vi "Angle_1.vi"() -> ()   [LabVIEW 2020]
uses:
  Support/Controls/Cmd_Mouse Popup.ctl
  Support/Controls/Clst_Initialize Input.ctl
  Support/Controls/Cmd_Var Data IO.ctl
  Variables/Global_Cal Info.vi
  Support/Public/Polymorph/Input Check_TBL.vi
  Support/Public/Polymorph/Input Check_TextBox.vi
panel:
  in  "반지름":string caption="투영면 반지름 (mm)"
  out "최소범위":string
  out "STD set":string[][](table) caption="○ 기준기 조합 (값)"
  in  "Measured 2":string[][](table)
  in  "표시방식":string(combo)
  out "단위":string
  out "최대범위":string
  in  "Spec 변경":bool
  in  "Random":bool
  out "Resolution":string[][](table) caption="Spec"
  out "Spec":string[][](table)
  out "제목":string
  out "에러 출력":errorcluster
  out "Condition":string[][](table) caption="2. 직선성 시험"
  in  "최소눈금":string(combo)
  in  "Measured":string[][](table) caption="저울의 지시값"
  out "Load?":bool
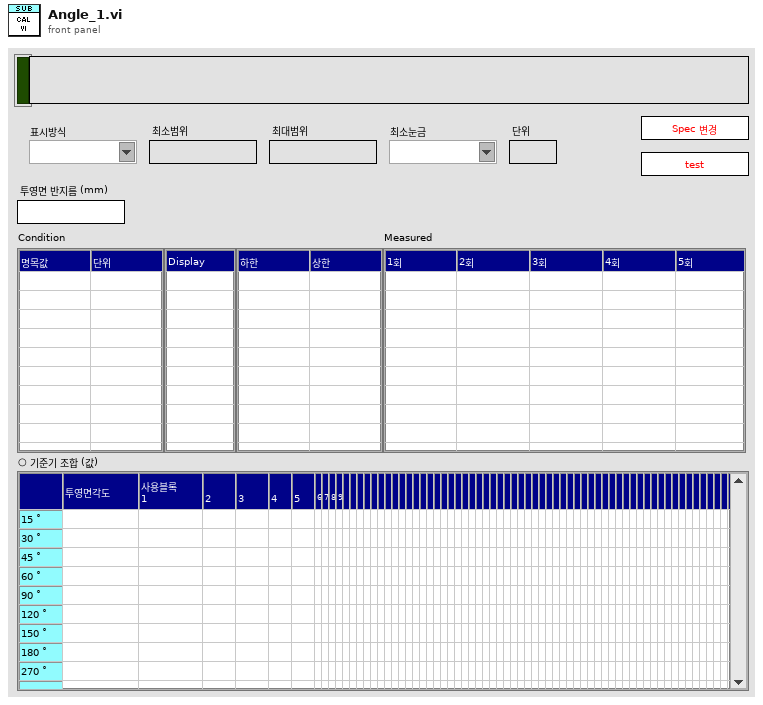
[diagram p1: front panel]
types:
  T1 = typedef "Cmd_Mouse Popup.ctl" = enum16{"활성화", "메뉴선택"}
  T2 = cluster{"Shift":bool, "Ctrl":bool, "Alt":bool, "Cmd":bool, "Opt":bool}
  T3 = typedef "Clst_Initialize Input.ctl" = cluster{"Initialize 1":cluster{"Condition":refnum<vi>[], "Spec":refnum<vi>[], "Measured":refnum<vi>[], "Resolution":refnum<vi>[], "Func_ext":string, "제목":refnum<vi>, "Measured_ADJ":refnum<vi>[]}, "Initialize 2":cluster{"문자열":refnum<vi>[], "콤보박스":refnum<vi>[], "링":refnum<vi>[], "열거형":refnum<vi>[], "테이블":refnum<vi>[], "여러열":refnum<vi>[], "디지털(DBL)":refnum<vi>[], "3D string":refnum<vi>[], "ctrl":refnum<vi>[], "boolean":refnum<vi>[]}}
  T4 = typedef "Cmd_Var Data IO.ctl" = enum16{"Condition", "Condition Default", "Condition_Temp", "Resolution", "Resolution Default", "Resolution Old", "Spec", "Spec Default", "Spec Old", "Spec Temp", "Result", "Result2", "Result3", "Result_Temp", "Result_ADJ", "Result_ADJ2", "STD1", "STD2", "STD3", "STD4", "STD5", "STD Temp", "CMC", "CMC Default"}
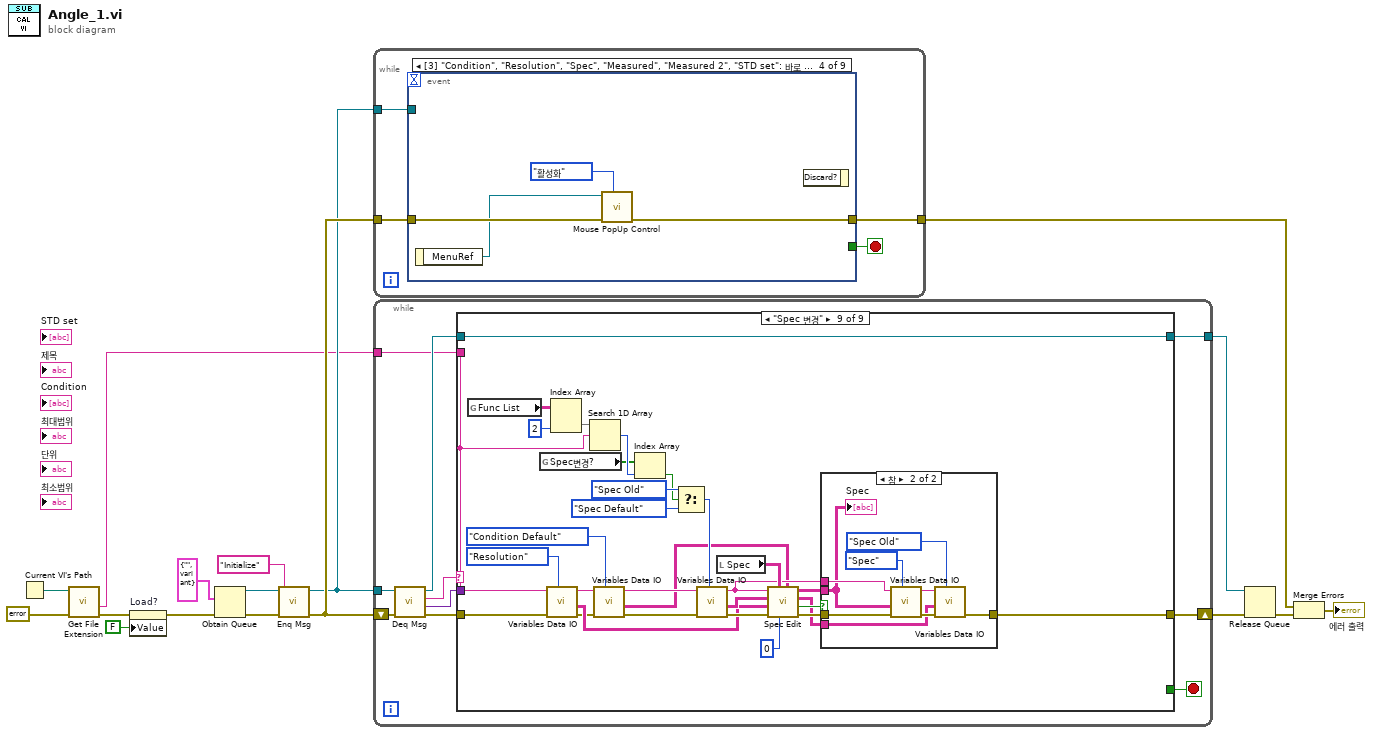
[diagram p0: block diagram]
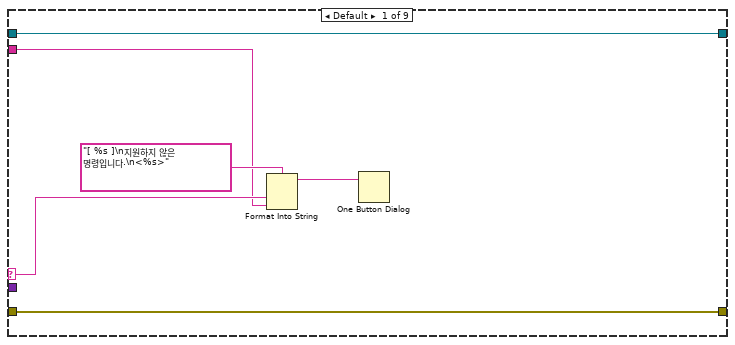
[diagram p2: hidden frame]
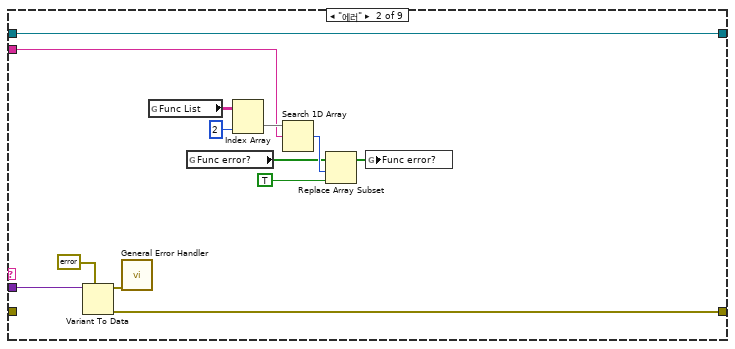
[diagram p3: hidden frame]
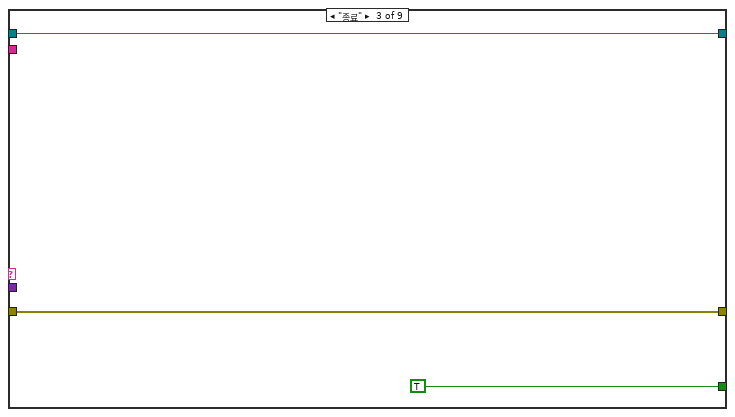
[diagram p4: hidden frame]
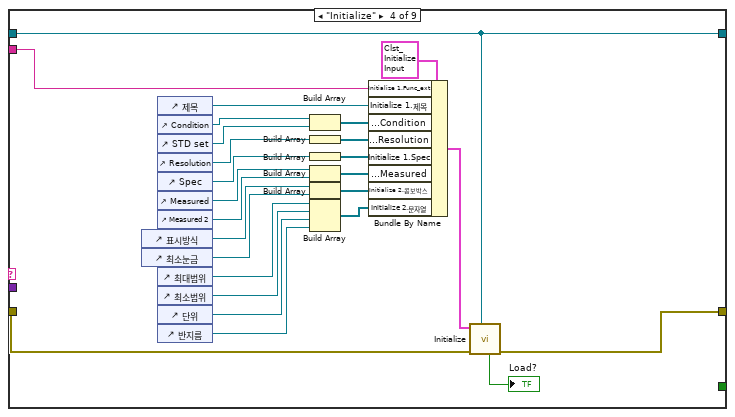
[diagram p5: hidden frame]
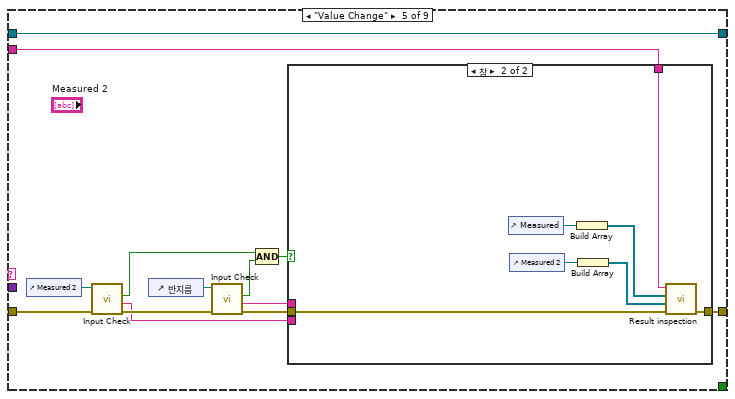
[diagram p6: hidden frame]
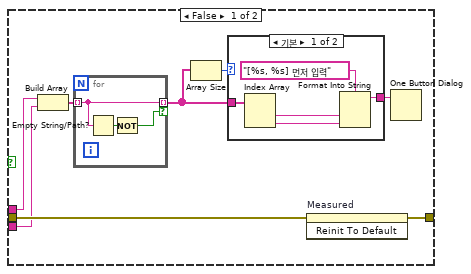
[diagram p7: hidden frame]
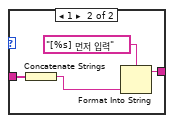
[diagram p8: hidden frame]
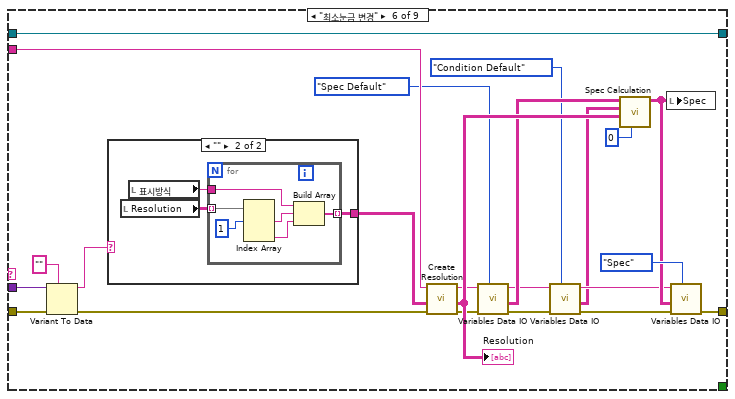
[diagram p9: hidden frame]
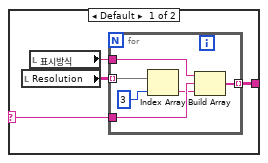
[diagram p10: hidden frame]
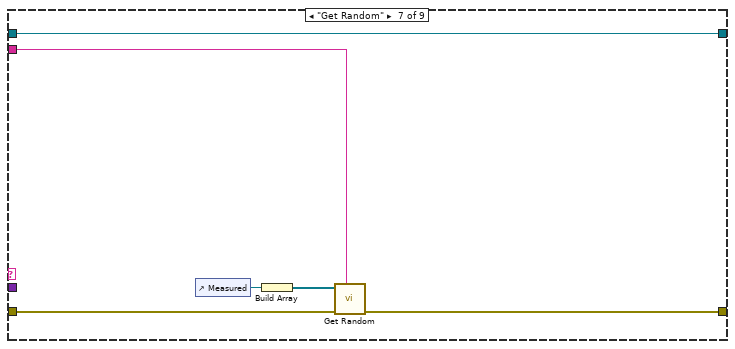
[diagram p11: hidden frame]
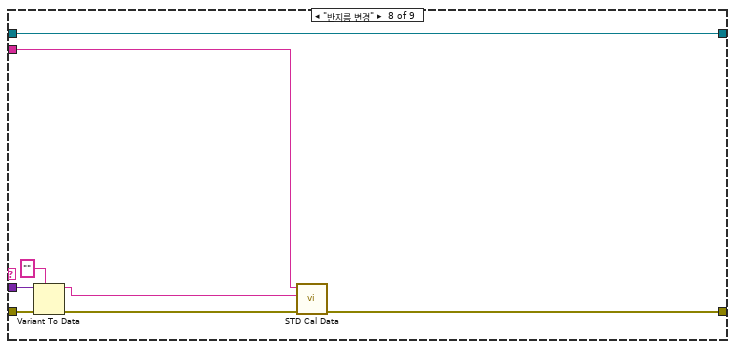
[diagram p12: hidden frame]
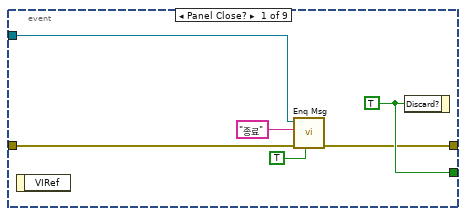
[diagram p14: hidden frame]
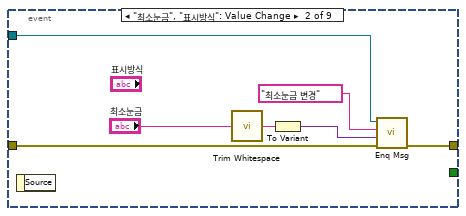
[diagram p15: hidden frame]
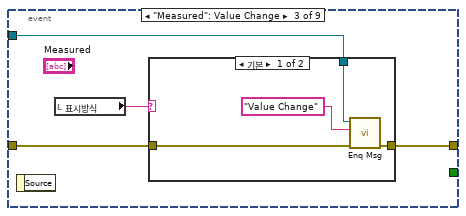
[diagram p16: hidden frame]
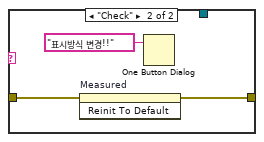
[diagram p17: hidden frame]
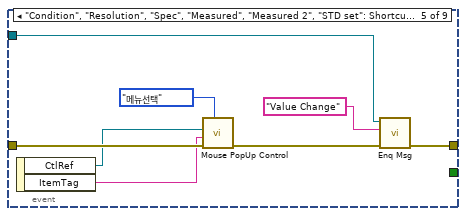
[diagram p18: hidden frame]
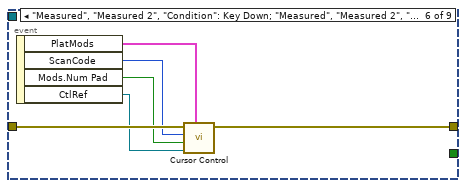
[diagram p19: hidden frame]
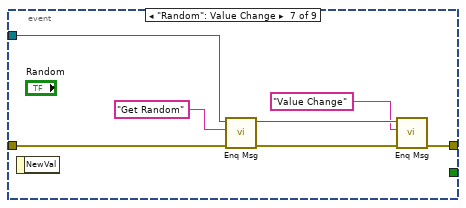
[diagram p20: hidden frame]
diagram:
  n1 = Current VI's Path() -> (path=w5:path)
  n2 = call <vilib>:"Get File Extension.vi"("error in (no error)"=errorcluster {"status"=FALSE, "code"=0, "source"=""} ("에러 상수"), "file"=w5) -> ("error out"=w3:errorcluster, "filename without extension"=w4:string)  [unwired: 5 in, 3 out]
  n3 = property on="Load?" class="Bool (엄격한)"(error in=w3, "Value"=FALSE ("Load?")) -> (error out=w2:errorcluster)  [unwired: 1 in, 1 out]
  n4 = Obtain Queue(element data type=cluster{"메세지":string, "값":variant} {"메세지"="", "값"=variant} ("Message Cluster"), error in (no error)=w2) -> (queue out=w14:refnum<queue>, error out=w16:errorcluster)  [unwired: 3 in, 1 out]
  n5 = call "Enq Msg.vi"("에러 입력(에러 없음)"=w16, "메세지"="Initialize", "큐 입력"=w14) -> ("에러 출력"=w15:errorcluster, "큐 출력"=w12:refnum<queue>)  [unwired: 7 in]
  n6 = while {
    tunnel: w15 -> [w19]
    tunnel: w12 -> [w20]
    tunnel: [w18] -> w9
    stop <- w21 stop-if-true
    n7 = event shown="[3] \"Condition\", \"Resolution\", \"Spec\", \"Measured\", \"Measured 2\", \"STD set\": 바로 가기 메뉴 활성화?" {
      selector: _ -> [_ _ _ _ _ _ _ _ _]
      dyn-events: _ -> [_ _ _ _ _ _ _ _ _]
      timeout: _ -> [_ _ _ _ _ _ _ _ _]
      tunnel: [w27 _ _ _ _ _ _ _ _] -> w21
      tunnel: w20 -> [w25 w33 w38 _ w50 _ w68 w72 w75]
      tunnel: w19 -> [w26 w34 w36 w49 w57 w63 w69 w73 w78]
      tunnel: [w23 w32 w37 w48 w51 w62 w64 w71 w77] -> w18
      event Panel Close? {
        w27 = TRUE ("버림?")
        n8 = event-data() -> ()  [unwired: 1 in, 1 out]
        n9 = call "Enq Msg.vi"("우선순위 메시지?"=TRUE, "에러 입력(에러 없음)"=w26, "메세지"="종료", "큐 입력"=w25) -> ("에러 출력"=w23:errorcluster)  [unwired: 6 in, 1 out]
        n10 = event-data("Discard?"=w27) -> ()  [unwired: 1 in, 1 out]
      }
      event "최소눈금", "표시방식": Value Change {
        n11 = event-data() -> ()  [unwired: 1 in, 1 out]
        n12 = call <vilib>:"Trim Whitespace.vi"("string"="최소눈금") -> ("trimmed string"=w30:string)  [unwired: 1 in]
        n13 = To Variant(anything=w30) -> (Variant=w28:variant)
        n14 = call "Enq Msg.vi"("에러 입력(에러 없음)"=w34, "값"=w28, "메세지"="최소눈금 변경", "큐 입력"=w33) -> ("에러 출력"=w32:errorcluster)  [unwired: 6 in, 1 out]
      }
      event "Measured": Value Change {
        n15 = event-data() -> ()  [unwired: 1 in, 1 out]
        n16 = local read "표시방식"() -> (w35:string)
        n17 = case shown="기본" w35 {
          tunnel: w38 -> [w42 _]
          tunnel: [w41 w43] -> w37
          tunnel: w36 -> [w40 w44]
          frame Default {
            n18 = call "Enq Msg.vi"("에러 입력(에러 없음)"=w40, "메세지"="Value Change", "큐 입력"=w42) -> ("에러 출력"=w41:errorcluster)  [unwired: 7 in, 1 out]
          }
          frame "Check" {
            n19 = invoke on="Measured" class="Tbl (엄격한)" method="Reinit To Default"(error in=w44) -> (error out=w43:errorcluster)  [unwired: 2 in, 2 out]
            n20 = One Button Dialog(message="표시방식 변경!!" ("메시지")) -> ()  [unwired: 1 in, 1 out]
          }
        }
      }
      event "Condition", "Resolution", "Spec", "Measured", "Measured 2", "STD set": Shortcut Menu Activation? {
        n21 = event-data() -> ("MenuRef"=w47:refnum<k9>)  [unwired: 1 in]
        n22 = call "Mouse PopUp Control.vi"("type"=Cmd_Mouse_Popup."활성화", "error in"=w49, "메뉴 참조"=w47) -> ("error out"=w48:errorcluster)  [unwired: 8 in]
        n23 = event-data() -> ()  [unwired: 2 in, 1 out]
      }
      event "Condition", "Resolution", "Spec", "Measured", "Measured 2", "STD set": Shortcut Menu Selection (User) {
        n24 = event-data() -> ("CtlRef"=w55:refnum<vi>, "ItemTag"=w54:string)  [unwired: 1 in]
        n25 = call "Mouse PopUp Control.vi"("type"=Cmd_Mouse_Popup."메뉴선택", "error in"=w57, "아이템 태그"=w54, "Tbl 참조 번호"=w55) -> ("error out"=w52:errorcluster)  [unwired: 7 in]
        n26 = call "Enq Msg.vi"("에러 입력(에러 없음)"=w52, "메세지"="Value Change", "큐 입력"=w50) -> ("에러 출력"=w51:errorcluster)  [unwired: 7 in, 1 out]
      }
      event "Measured", "Measured 2", "Condition": Key Down; "Measured", "Measured 2", "Condition": Key Repeat {
        n27 = event-data() -> ("PlatMods"=w58:T2, "ScanCode"=w61:i16, "Mods.Num Pad"=w60:bool, "CtlRef"=w59:refnum<vi>)  [unwired: 1 in]
        n28 = call "Cursor Control.vi"("플랫폼 조합키"=w58, "참조"=w59, "Num Pad"=w60, "ScanCode"=w61, "error in"=w63) -> ("error out"=w62:errorcluster)  [unwired: 5 in, 1 out]
      }
      event "Random": Value Change {
        n29 = event-data() -> ()  [unwired: 1 in, 1 out]
        n30 = call "Enq Msg.vi"("에러 입력(에러 없음)"=w69, "메세지"="Get Random", "큐 입력"=w68) -> ("에러 출력"=w67:errorcluster, "큐 출력"=w66:refnum<queue>)  [unwired: 7 in]
        n31 = call "Enq Msg.vi"("에러 입력(에러 없음)"=w67, "메세지"="Value Change", "큐 입력"=w66) -> ("에러 출력"=w64:errorcluster)  [unwired: 7 in, 1 out]
      }
      event "Spec 변경": Value Change {
        n32 = event-data() -> ()  [unwired: 1 in, 1 out]
        n33 = call "Enq Msg.vi"("에러 입력(에러 없음)"=w73, "메세지"="Spec 변경", "큐 입력"=w72) -> ("에러 출력"=w71:errorcluster)  [unwired: 7 in, 1 out]
      }
      event "반지름": Value Change {
        n34 = event-data() -> ()  [unwired: 1 in, 2 out]
        n35 = To Variant(anything="반지름") -> (Variant=w80:variant)
        n36 = call "Enq Msg.vi"("에러 입력(에러 없음)"=w78, "값"=w80, "메세지"="반지름 변경", "큐 입력"=w75) -> ("에러 출력"=w77:errorcluster)  [unwired: 6 in, 1 out]
      }
    }
  }
  n37 = while {
    shift-right: [w90] -> w11
    shift-left: w15 -> [w89]
    tunnel: w12 -> [w87]
    tunnel: [w82] -> w10
    tunnel: w4 -> [w81]
    stop <- w83 stop-if-true
    n38 = call "Deq Msg.vi"("에러 입력(에러 없음)"=w89, "큐 입력"=w87) -> ("에러 출력"=w88:errorcluster, "값"=w84:variant, "메세지"=w86:string, "큐 출력"=w85:refnum<queue>)  [unwired: 6 in]
    n39 = case shown="\"Spec 변경\"" w86 {
      selector: w86 -> [w92 _ _ _ _ _ _ _ _]
      tunnel: w88 -> [w96 _ w112 w138 w148 w200 w222 w229 w257]
      tunnel: [w96 w106 w112 w116 w150 w193 w223 w227 w260] -> w90
      tunnel: w85 -> [w95 w105 w110 w123 w151 w201 w226 w234 w264]
      tunnel: w84 -> [_ w107 _ _ _ w199 _ w230 _]
      tunnel: [_ _ TRUE ("버림?") _ _ _ _ _ _] -> w83
      tunnel: [w95 w105 w110 w123 w151 w201 w226 w234 w264] -> w82
      tunnel: w81 -> [w91 w97 _ w124 w149 w197 w221 w228 w242]
      frame Default {
        n40 = Format Into String(format string="[ %s ]\n지원하지 않은 명령입니다.\n<%s>" ("메시지"), w92, w91) -> (resulting string=w93:string)  [unwired: 2 in, 1 out]
        n41 = One Button Dialog(message=w93) -> ()  [unwired: 1 in, 1 out]
      }
      frame "에러" {
        n42 = Variant To Data(type=errorcluster {"status"=FALSE, "code"=0, "source"=""} ("에러 출력"), Variant=w107) -> (data=w109:errorcluster, error out=w106:errorcluster)  [unwired: 1 in]
        n43 = call <vilib>:"General Error Handler.vi"("error in (no error)"=w109) -> ()  [unwired: 10 in, 5 out]
        n44 = global read "Global_Cal Info.vi" "Func List"() -> (w99:string[][])
        n45 = global read "Global_Cal Info.vi" "Func error?"() -> (w102:bool[])
        n46 = Index Array(array=w99, index (col)=2 ("비활성화된 인덱스 (열)")) -> (element=w100:string[])  [unwired: 1 in]
        n47 = Search 1D Array(1D array=w100, element=w97) -> (index of element=w103:i32)  [unwired: 1 in]
        n48 = Replace Array Subset(array=w102, new element=TRUE ("새 원소/부분배열"), index=w103) -> (w104:bool[])
        n49 = global write "Global_Cal Info.vi" "Func error?"(w104) -> ()
      }
      frame "종료" {
      }
      frame "Initialize" {
        n50 = control-ref of="표시방식"() -> (w122:refnum<vi>)
        n51 = control-ref of="최소눈금"() -> (w131:refnum<vi>)
        n52 = control-ref of="제목"() -> (w129:refnum<vi>)
        n53 = control-ref of="Condition"() -> (w135:refnum<vi>)
        n54 = control-ref of="STD set"() -> (w117:refnum<vi>)
        n55 = control-ref of="Resolution"() -> (w125:refnum<vi>)
        n56 = control-ref of="Spec"() -> (w128:refnum<vi>)
        n57 = control-ref of="Measured"() -> (w132:refnum<vi>)
        n58 = control-ref of="Measured 2"() -> (w118:refnum<vi>)
        n59 = control-ref of="최대범위"() -> (w115:refnum<vi>)
        n60 = control-ref of="최소범위"() -> (w119:refnum<vi>)
        n61 = control-ref of="단위"() -> (w121:refnum<vi>)
        n62 = control-ref of="반지름"() -> (w113:refnum<vi>)
        n63 = Build Array(w135, w117) -> (w134:refnum<vi>[])
        n64 = Build Array(w125) -> (w126:refnum<vi>[])
        n65 = Build Array(w128) -> (w127:refnum<vi>[])
        n66 = Build Array(w132, w118) -> (w133:refnum<vi>[])
        n67 = Build Array(w122, w131) -> (w130:refnum<vi>[])
        n68 = Build Array(w115, w119, w121, w113) -> (w120:refnum<vi>[])
        n69 = Bundle By Name(cluster=T3 {"Initialize 1"={"Condition"=[], "Spec"=[], "Measured"=[], "Resolution"=[], "Func_ext"="", "제목"=refnum, "Measured_ADJ"=[]}, "Initialize 2"={"문자열"=[], "콤보박스"=[], "링"=[], "열거형"=[], "테이블"=[], "여러열"=[], "디지털(DBL)"=[], "3D string"=[], "ctrl"=[], "boolean"=[]}} ("입력 클러스터"), "Initialize 1.Func_ext"=w124, "Initialize 1.제목"=w129, "Initialize 1.Condition"=w134, "Initialize 1.Resolution"=w126, "Initialize 1.Spec"=w127, "Initialize 1.Measured"=w133, "Initialize 2.콤보박스"=w130, "Initialize 2.문자열"=w120) -> (w136:T3)
        n70 = call "Initialize.vi"("큐 입력"=w123, "error in"=w138, "입력 클러스터"=w136) -> ("error out"=w116:errorcluster, "Load?"=→"Load?":bool)  [unwired: 5 in, 2 out]
      }
      frame "Value Change" {
        n71 = control-ref of="Measured 2"() -> (w144:refnum<vi>)
        n72 = call-poly "Input Check.vi"("에러 입력"=w148, "Table 참조"=w144) -> ("에러 출력"=w146:errorcluster, "Caption.Text"=w142:string, "내용있음?"=w140:bool)  [unwired: 6 in, 1 out]
        n73 = control-ref of="반지름"() -> (w143:refnum<vi>)
        n74 = call-poly "Input Check.vi"("에러 입력"=w146, "TextBox 참조"=w143) -> ("에러 출력"=w145:errorcluster, "Caption.Text"=w141:string, "내용있음?"=w139:bool)  [unwired: 7 in]
        n75 = Compound Arithmetic op=AND ("복합 연산")(w140, w139) -> (w147:bool)
        n76 = case shown="참" w147 {
          tunnel: [w158 w178] -> w150
          tunnel: w149 -> [_ w177]
          tunnel: w145 -> [w159 w174]
          tunnel: w141 -> [w155 _]
          tunnel: w142 -> [w154 _]
          frame False {
            n77 = Build Array(w155, w154) -> (w153:string[])
            n78 = for {
              tunnel: w153 -> [w162] mode=indexing
              tunnel: [w162] -> w152 mode=indexing if=w160
              n79 = Empty String/Path?(string/path=w162) -> (empty?=w161:bool)
              n80 = Not(x=w161) -> (.not. x?=w160:bool)
            }
            n81 = Array Size(array=w152) -> (size(s)=w156:i32)
            n82 = case shown="기본" w156 {
              tunnel: [w166 w170] -> w157
              tunnel: w152 -> [w165 w169]
              frame Default {
                n83 = Index Array(array=w165) -> (element #1=w164:string, element #2=w163:string)  [unwired: 2 in]
                n84 = Format Into String(format string="[%s, %s] 먼저 입력" ("포맷 문자열"), w164, w163) -> (resulting string=w166:string)  [unwired: 2 in, 1 out]
              }
              frame 1 {
                n85 = Concatenate Strings(w169) -> (w168:string)
                n86 = Format Into String(format string="[%s] 먼저 입력" ("포맷 문자열"), w168) -> (resulting string=w170:string)  [unwired: 2 in, 1 out]
              }
            }
            n87 = invoke on="Measured" class="Tbl (엄격한)" method="Reinit To Default"(error in=w159) -> (error out=w158:errorcluster)  [unwired: 2 in, 2 out]
            n88 = One Button Dialog(message=w157) -> ()  [unwired: 1 in, 1 out]
          }
          frame True {
            n89 = control-ref of="Measured"() -> (w176:refnum<vi>)
            n90 = control-ref of="Measured 2"() -> (w173:refnum<vi>)
            n91 = Build Array(w176) -> (w175:refnum<vi>[])
            n92 = Build Array(w173) -> (w172:refnum<vi>[])
            n93 = call "Result inspection.vi"("error in"=w174, "Ref. Data (excluded)"=w172, "Ref. Data (Inspection)"=w175, "Func ext"=w177) -> ("error out"=w178:errorcluster)  [unwired: 4 in, 3 out]
          }
        }
      }
      frame "최소눈금 변경" {
        n94 = Variant To Data(error in=w200, type="", Variant=w199) -> (data=w186:string, error out=w188:errorcluster)
        n95 = case shown="\"\"" w186 {
          selector: w186 -> [w202 _]
          tunnel: [w205 w214] -> w187
          frame Default {
            n96 = local read "Resolution"() -> (w204:string[][])
            n97 = local read "표시방식"() -> (w203:string)
            n98 = for {
              tunnel: w204 -> [w211] mode=indexing
              tunnel: w202 -> [w210]
              tunnel: [w208] -> w205 mode=indexing
              tunnel: w203 -> [w207]
              n99 = Index Array(array=w211, index=3 ("인덱스")) -> (element=w209:string)
              n100 = Build Array(w207, w210, w209) -> (w208:string[])
            }
          }
          frame "" {
            n101 = local read "Resolution"() -> (w213:string[][])
            n102 = local read "표시방식"() -> (w212:string)
            n103 = for {
              tunnel: w213 -> [w220] mode=indexing
              tunnel: [w219] -> w214 mode=indexing
              tunnel: w212 -> [w218]
              n104 = Index Array(array=w220, index #1=1 ("인덱스")) -> (element #1=w216:string, element #3=w215:string)  [unwired: 2 in, 1 out]
              n105 = Build Array(w218, w216, w215) -> (w219:string[])
            }
          }
        }
        n106 = call "Create Resolution.vi"("에러 입력(에러 없음)"=w188, "Resolution"=w187, "Func_ext"=w197) -> ("에러 출력"=w191:errorcluster, "Resolution Out"=w194:string[][], "Func_ext 출력"=w190:string)  [unwired: 6 in]
        "Resolution" <- w194
        n107 = call "Variables Data IO.vi"("Select"=Cmd_Var_Data_IO."Spec Default", "error in"=w191, "Func_ext"=w190) -> ("error out"=w182:errorcluster, "Data Out"=w189:string[][], "Func_ext Out"=w183:string)  [unwired: 6 in]
        n108 = call "Variables Data IO.vi"("Select"=Cmd_Var_Data_IO."Condition Default", "error in"=w182, "Func_ext"=w183) -> ("error out"=w180:errorcluster, "Data Out"=w179:string[][], "Func_ext Out"=w181:string)  [unwired: 6 in]
        n109 = call "Spec Calculation.vi"("기준값 열번호"=0 ("열번호(기준값)"), "Resolution"=w194, "Condition in"=w179, "Spec Default"=w189) -> ("Spec out"=w185:string[][])  [unwired: 6 in, 1 out]
        n110 = local write "Spec"(w185) -> ()
        n111 = call "Variables Data IO.vi"("Select"=Cmd_Var_Data_IO."Spec", "error in"=w180, "Data In"=w185, "Func_ext"=w181) -> ("error out"=w193:errorcluster)  [unwired: 5 in, 2 out]
      }
      frame "Get Random" {
        n112 = control-ref of="Measured"() -> (w225:refnum<vi>)
        n113 = Build Array(w225) -> (w224:refnum<vi>[])
        n114 = call "Get Random.vi"("Func_Ext"=w221, "에러 입력"=w222, "Meas"=w224) -> ("에러 출력"=w223:errorcluster)  [unwired: 7 in, 1 out]
      }
      frame "반지름 변경" {
        n115 = Variant To Data(error in=w229, type="", Variant=w230) -> (data=w233:string, error out=w231:errorcluster)
        n116 = call "STD Cal Data.vi"("error in"=w231, "문자열"=w233, "Func_ext"=w228) -> ("error out"=w227:errorcluster)  [unwired: 4 in, 4 out]
      }
      frame "Spec 변경" {
        n117 = global read "Global_Cal Info.vi" "Func List"() -> (w247:string[][])
        n118 = global read "Global_Cal Info.vi" "Spec변경?"() -> (w243:bool[])
        n119 = call "Variables Data IO.vi"("Select"=Cmd_Var_Data_IO."Resolution", "error in"=w257, "Func_ext"=w242) -> ("error out"=w240:errorcluster, "Data Out"=w251:string[][], "Func_ext Out"=w238:string)  [unwired: 6 in]
        n120 = Index Array(array=w247, index (col)=2 ("비활성화된 인덱스 (열)")) -> (element=w245:string[])  [unwired: 1 in]
        n121 = Search 1D Array(1D array=w245, element=w242) -> (index of element=w244:i32)  [unwired: 1 in]
        n122 = call "Variables Data IO.vi"("Select"=Cmd_Var_Data_IO."Condition Default", "error in"=w240, "Func_ext"=w238) -> ("error out"=w239:errorcluster, "Data Out"=w235:string[][], "Func_ext Out"=w237:string)  [unwired: 6 in]
        n123 = Index Array(array=w243, index=w244) -> (element=w248:bool)
        n124 = Select(t=Cmd_Var_Data_IO."Spec Old" ("Select"), s=w248, f=Cmd_Var_Data_IO."Spec Default" ("Select")) -> (s? t:f=w241:T4)
        n125 = call "Variables Data IO.vi"("Select"=w241, "error in"=w239, "Func_ext"=w237) -> ("error out"=w259:errorcluster, "Data Out"=w252:string[][], "Func_ext Out"=w253:string)  [unwired: 6 in]
        n126 = local read "Spec"() -> (w254:string[][])
        n127 = call "Spec Edit.vi"("Condition"=w235, "열번호(기준값)"=0, "Spec Value"=w254, "에러 입력(에러 없음)"=w259, "Resolution"=w251, "Spec Default"=w252, "Func_ext"=w253) -> ("에러 출력"=w261:errorcluster, "변경?"=w262:bool, "Spec Default out"=w256:string[][], "Spec 출력"=w263:string[][])  [unwired: 1 in]
        n128 = case shown="참" w262 {
          tunnel: w263 -> [_ w271]
          tunnel: w261 -> [w265 w274]
          tunnel: [w265 w269] -> w260
          tunnel: w253 -> [_ w272]
          tunnel: w256 -> [_ w267]
          frame False {
          }
          frame True {
            n129 = call "Variables Data IO.vi"("Select"=Cmd_Var_Data_IO."Spec", "error in"=w274, "Data In"=w271, "Func_ext"=w272) -> ("error out"=w270:errorcluster, "Func_ext Out"=w268:string)  [unwired: 5 in, 1 out]
            n130 = call "Variables Data IO.vi"("Select"=Cmd_Var_Data_IO."Spec Old", "error in"=w270, "Data In"=w267, "Func_ext"=w268) -> ("error out"=w269:errorcluster)  [unwired: 5 in, 2 out]
            "Spec" <- w271
          }
        }
      }
    }
  }
  n131 = Release Queue(queue=w10, error in (no error)=w11) -> (error out=w8:errorcluster)  [unwired: 1 in, 2 out]
  n132 = Merge Errors(w9, w8) -> (→"에러 출력":errorcluster)
